vi "Method_Const.vi"(4 "Value":i32, 5 "Value A":refnum<class "Abs_I32 Integer.lvclass">) -> (1 "Result":refnum<class "Abs_Boolean.lvclass">)   [LabVIEW 2021, in "Equal_I32.lvclass"]
uses:
  Equal_I32.lvclass
  Abs_Types/I32 Integer/Abs_I32 Integer.lvclass
  C:/Program Files (x86)/National Instruments/LabVIEW 2021/vi.lib/TSA/Abstract Data Classes/Abs_Types/Numeric/Abs_Numeric.lvclass
  Abs_Types/Boolean/Abs_Boolean.lvclass
  C:/TSA/LV_Abstract/Source/Functions/Support/Compare/Two Term/I32/AbsComp_Two Term_I32.lvclass
  C:/Program Files (x86)/National Instruments/LabVIEW 2021/vi.lib/TSA/Abstract Data Classes/Abs_Types/Boolean/Abs_Boolean.lvclass
  Support/Compare/Two Term/I32/AbsComp_Two Term_I32.lvclass/AbsComp_Two Term_I32.ctl
  Support/Compare/Two Term/I32/Properties/Write Numeric A.vi
  Support/Compare/Two Term/I32/Properties/Write Numeric B.vi
  Constants/Support/I32/Const_I32.lvclass
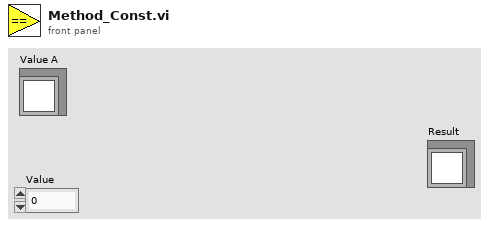
[diagram p1: front panel]
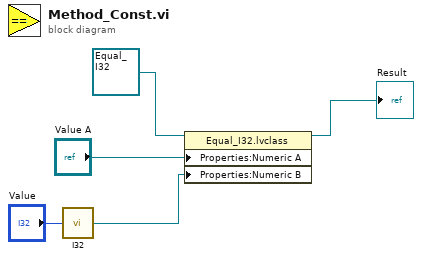
[diagram p0: block diagram]
diagram:
  n1 = call "I32.vi"("Value"="Value") -> ("Constant"=w2:refnum<class "Abs_I32 Integer.lvclass">)  [unwired: 4 in]
  n2 = property class="Equal_I32.lvclass"(reference=refnum<class "Equal_I32.lvclass"> refnum ("Greater 0_U64.lvclass"), "Properties:Numeric A"="Value A", "Properties:Numeric B"=w2) -> (reference out=→"Result":refnum<class "Equal_I32.lvclass">)  [unwired: 1 in, 1 out]
